vi "displayerrors.vi"() -> (0 "error IO":errorcluster)   [LabVIEW 2015]
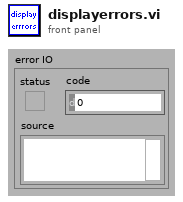
[diagram p1: front panel]
types:
  T1 = cluster{"AO":refnum<k21>[], "E_AO":errorcluster[]}
  T2 = cluster{" AI":refnum<k21>, "E_AI":errorcluster, "header":dbl[]}
  T3 = cluster{"CI":refnum<k21>[], "E_CI":errorcluster[]}
  T4 = cluster{"filetif":refnum<file>[], "E_filetif":errorcluster[]}
  T5 = cluster{"E_binfile":errorcluster[], "binfile":refnum<file>[]}
  T6 = cluster{"upleft":bool, "up":bool, "upright":bool, "right":bool, "downright":bool, "down":bool, "downleft":bool, "left":bool, "Bigsmall":bool, "E_stage":errorcluster}
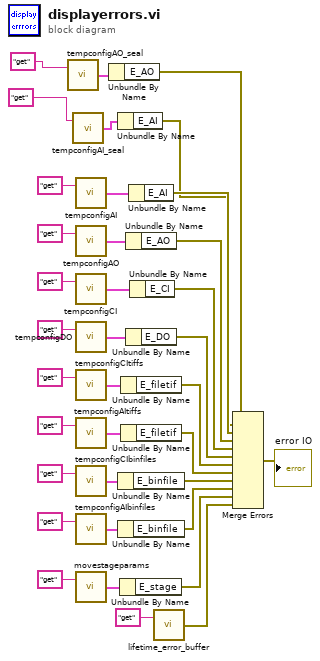
[diagram p0: block diagram]
diagram:
  n1 = call "tempconfigAO_seal.vi"("command"="get") -> ("Temp Config out"=w4:T1)  [unwired: 1 in]
  n2 = call "tempconfigAI_seal.vi"("command"="get") -> ("Temp Config out"=w3:T2)  [unwired: 1 in]
  n3 = call "tempconfigAI.vi"("command"="get") -> ("Temp Config out"=w30:T2)  [unwired: 1 in]
  n4 = call "tempconfigAO.vi"("command"="get") -> ("Temp Config out"=w31:T1)  [unwired: 1 in]
  n5 = call "tempconfigCI.vi"("command"="get") -> ("Temp Config out"=w19:T3)  [unwired: 1 in]
  n6 = call "tempconfigDO.vi"("command"="get") -> ("Temp Config out"=w32:cluster{"DO":refnum<k21>, "E_DO":errorcluster})  [unwired: 1 in]
  n7 = call "tempconfigCItiffs.vi"("command"="get") -> ("Temp Config out"=w21:T4)  [unwired: 1 in]
  n8 = call "tempconfigAItiffs.vi"("command"="get") -> ("Temp Config out"=w23:T4)  [unwired: 1 in]
  n9 = call "tempconfigCIbinfiles.vi"("command"="get") -> ("Temp Config out"=w13:T5)  [unwired: 1 in]
  n10 = call "tempconfigAIbinfiles.vi"("command"="get") -> ("Temp Config out"=w12:T5)  [unwired: 1 in]
  n11 = call "movestageparams.vi"("command"="get") -> ("Params out"=w25:T6)  [unwired: 1 in]
  n12 = Unbundle By Name(w4) -> ("E_AO"=w2:errorcluster[])
  n13 = Unbundle By Name(w3) -> ("E_AI"=w1:errorcluster)
  n14 = Unbundle By Name(w13) -> ("E_binfile"=w11:errorcluster[])
  n15 = Unbundle By Name(w12) -> ("E_binfile"=w10:errorcluster[])
  n16 = Unbundle By Name(w25) -> ("E_stage"=w8:errorcluster)
  n17 = Unbundle By Name(w21) -> ("E_filetif"=w17:errorcluster[])
  n18 = Unbundle By Name(w23) -> ("E_filetif"=w16:errorcluster[])
  n19 = Unbundle By Name(w31) -> ("E_AO"=w34:errorcluster[])
  n20 = Unbundle By Name(w32) -> ("E_DO"=w35:errorcluster)
  n21 = Unbundle By Name(w30) -> ("E_AI"=w33:errorcluster)
  n22 = Unbundle By Name(w19) -> ("E_CI"=w18:errorcluster[])
  n23 = call "lifetime_error_buffer.vi"("command"="get") -> ("error out"=w7:errorcluster)  [unwired: 1 in]
  n24 = Merge Errors(w2, w1, w33, w34, w18, w35, w17, w16, w11, w10, w8, w7) -> (→"error IO":errorcluster)
